vi "LS336_read_temperature.vi"(0 "VISA Refnum in":refnum<visa-resource-name>, 1 "Setpoint (0.00000)":dbl format="%.5f", 2 "Gain (P) (50.0)":dbl=50.0 format="%.1f", 3 "Ramp Rate (0.0)":dbl format="%.1f", 4 "Max Current (0:User Specified)":u16(ring) items=["User Specified", "0.707 A", "1.0 A", "1.141 A", "2.0 A"], 5 "Setpoint Ramping \nEnable (F: Off)":bool, 6 "Heater Out Display (1:Current)":u16(ring)=1 items=["Current"=1, "Power"=2], 8 "Input (0:None)":u16(ring) items=["None", "A", "B", "C", "D"], 9 "Reset (I) (20.0)":dbl=20.0 format="%.1f", 10 "Mode (0:Off)":u16(ring) items=["Off", "Closed Loop PID", "Zone", "Open Loop"], 11 "Max User Current (2.000)":dbl=2.0 format="%.3f", 12 "Output's Control Loop (1:1)":u16(ring)=1 items=["1"=1, "2"=2], 13 "Rate (D) (0.0 %)":dbl format="%.1f", 14 "Power Up Enable (F: Off)":bool, 15 "Heater Resistance (1:25 Ohms)":u16(ring)=1 items=["25 Ohms"=1, "50 Ohms"=2], 16 "Manual Output (0.00 %)":dbl format="%.2f", 17 "Enable Setpoint (F:Off)":bool, 18 "Range (0:Off)":u16(ring) items=["Off", "Low (On)", "Medium", "High"]) -> (20 "VISA Refnum out":refnum<visa-resource-name>, 27 "error out":errorcluster)   [LabVIEW 2017]
uses:
  <instrlib>/Lake Shore 336/Lake Shore 336.lvlib
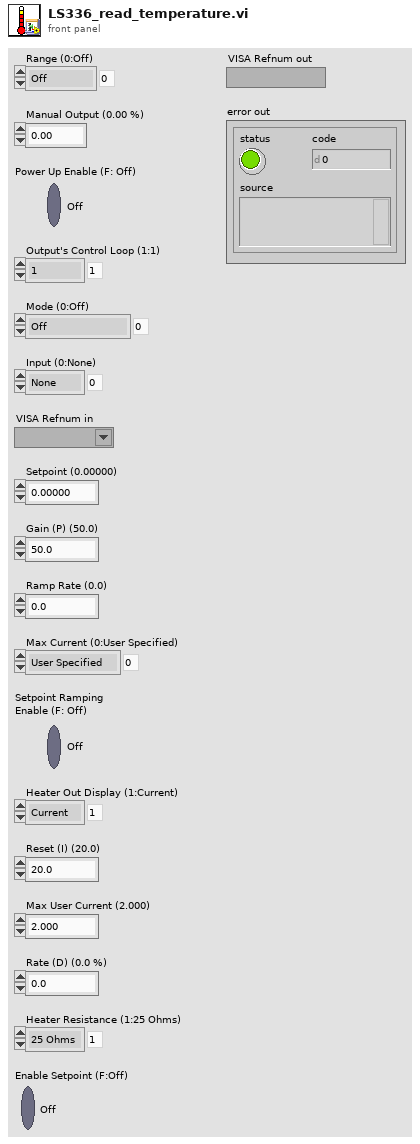
[diagram p1: front panel]
types:
  T1 = cluster{"Baud Rate":u32, "Parity":u16, "Data Bits":u16, "Stop Bits":u16, "Flow Control":u16}
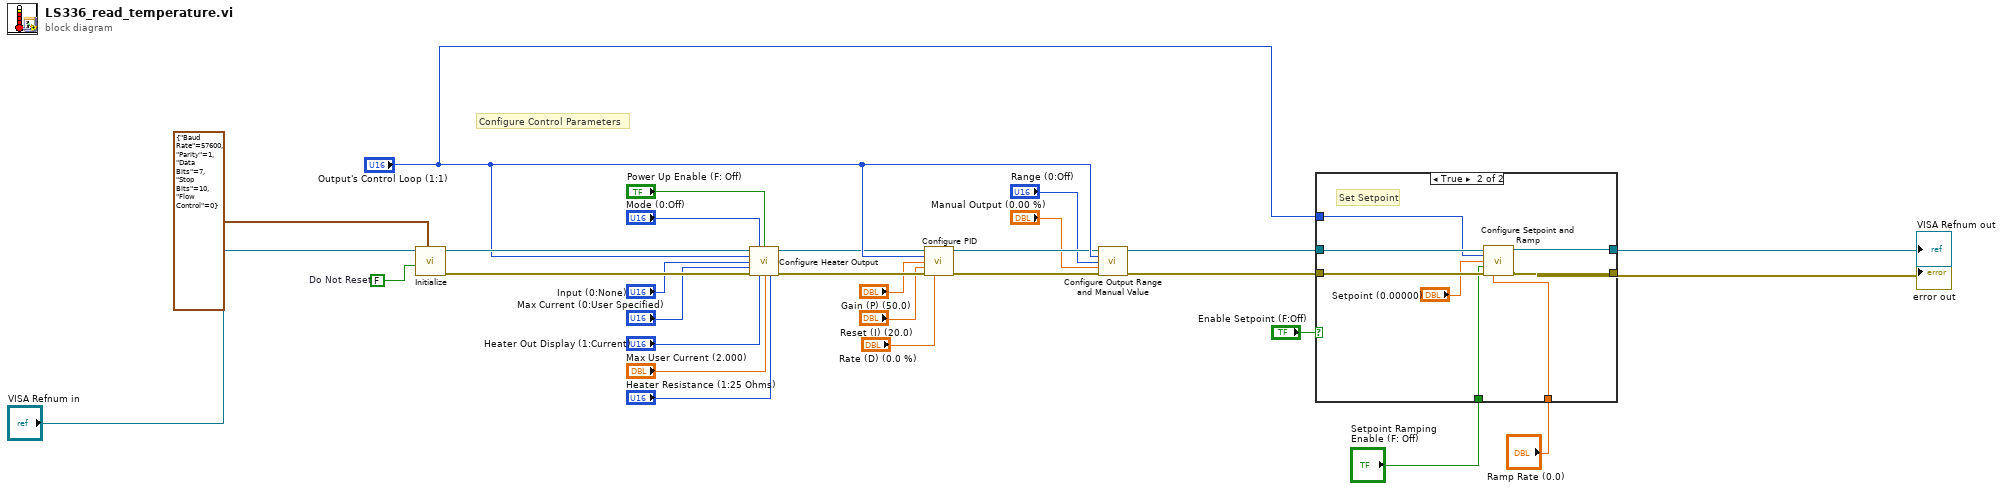
[diagram p0: block diagram]
diagram:
  w21 = FALSE  # Do Not Reset
  # "Configure Control Parameters"
  n1 = call <instrlib>:"Initialize.vi"("Serial Configuration"=T1 {"Baud Rate"=57600, "Parity"=1, "Data Bits"=7, "Stop Bits"=10, "Flow Control"=0}, "Reset (True)"=w21, "VISA resource name"="VISA Refnum in") -> ("error out"=w26:errorcluster, "VISA resource name out"=w27:refnum<visa-resource-name>)  [unwired: 7 in]
  n2 = call <instrlib>:"Configure Heater Output.vi"("VISA resource name"=w27, "Mode (0:Off)"="Mode (0:Off)", "Power Up Enable (F: Off)"="Power Up Enable (F: Off)", "Heater Output (1:1)"="Output's Control Loop (1:1)", "Input (0:None)"="Input (0:None)", "Max Current (0:User Specified)"="Max Current (0:User Specified)", "error in (no error)"=w26, "Heater Out Display (1:Current)"="Heater Out Display (1:Current)", "Max User Current (2.000)"="Max User Current (2.000)", "Heater Resistance (1:25 Ohms)"="Heater Resistance (1:25 Ohms)") -> ("VISA resource name out"=w17:refnum<visa-resource-name>, "error out"=w18:errorcluster)  [unwired: 4 in]
  n3 = call <instrlib>:"Configure PID.vi"("VISA resource name"=w17, "Output's Control Loop (1:1)"="Output's Control Loop (1:1)", "Gain (P) (50.0)"="Gain (P) (50.0)", "Reset (I) (20.0)"="Reset (I) (20.0)", "error in (no error)"=w18, "Rate (D) (0.0 %)"="Rate (D) (0.0 %)") -> ("VISA resource name out"=w16:refnum<visa-resource-name>, "error out"=w15:errorcluster)  [unwired: 8 in]
  n4 = call <instrlib>:"Configure Output Range and Manual Value.vi"("VISA resource name"=w16, "Output (1:1)"="Output's Control Loop (1:1)", "Range (0:Off)"="Range (0:Off)", "Manual Output (0.00 %)"="Manual Output (0.00 %)", "error in (no error)"=w15) -> ("VISA resource name out"=w23:refnum<visa-resource-name>, "error out"=w22:errorcluster)  [unwired: 9 in]
  n5 = case shown="True" "Enable Setpoint (F:Off)" {
    tunnel: "Output's Control Loop (1:1)" -> [_ w37]
    tunnel: w23 -> [w31 w38]
    tunnel: w22 -> [w30 w39]
    tunnel: [w30 w34] -> w1
    tunnel: [w31 w35] -> w2
    tunnel: "Setpoint Ramping \nEnable (F: Off)" -> [_ w33]
    tunnel: "Ramp Rate (0.0)" -> [_ w32]
    frame False {
      # "Do Not Set Setpoint"
    }
    frame True {
      # "Set Setpoint"
      n6 = call <instrlib>:"Configure Setpoint and Ramp.vi"("VISA resource name"=w38, "Output's Control Loop (1:1)"=w37, "Setpoint (0.00000)"="Setpoint (0.00000)", "Setpoint Ramping \nEnable (F: Off)"=w33, "error in (no error)"=w39, "Ramp Rate (0.0)"=w32) -> ("VISA resource name out"=w35:refnum<visa-resource-name>, "error out"=w34:errorcluster)  [unwired: 8 in]
    }
  }
  "VISA Refnum out" <- w2
  "error out" <- w1
